vi "Get Visible (Label).vi"(8 "error in (no error)":errorcluster, 10 "Label":string, 11 "IObject in":refnum<class "IObject.lvclass">) -> (0 "error out":errorcluster, 1 "Match?":bool, 2 "Visible?":bool, 3 "IObject out":refnum<class "IObject.lvclass">, 4 "Item visible?":bool)   [LabVIEW 2021, in "IObject.lvclass"]
uses:
  IObject.lvclass
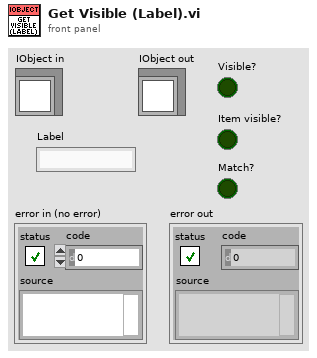
[diagram p1: front panel]
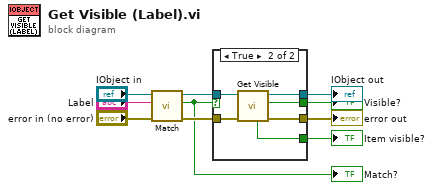
[diagram p0: block diagram]
diagram:
  n1 = call "Match.vi"("error in (no error)"="error in (no error)", "Label"="Label", "MMI Scaling in"="IObject in") -> ("error out"=w7:errorcluster, "Match?"=w1:bool, "MMI Scaling out"=w5:refnum<class "IObject.lvclass">)  [unwired: 6 in]
  "Match?" <- w1
  n2 = case shown="True" w1 {
    tunnel: w7 -> [w11 w18]
    tunnel: [w11 w17] -> w6
    tunnel: w5 -> [w12 w16]
    tunnel: [w12 w15] -> w4
    tunnel: [_ w14] -> w3
    tunnel: [_ w13] -> w2
    frame False {
    }
    frame True {
      n3 = call-dynamic "Get Visible.vi"("error in (no error)"=w18, "IObject in"=w16) -> ("error out"=w17:errorcluster, "Visible?"=w14:bool, "IObject out"=w15:refnum<class "IObject.lvclass">, "Item visible?"=w13:bool)  [unwired: 6 in]
    }
  }
  "error out" <- w6
  "IObject out" <- w4
  "Visible?" <- w3
  "Item visible?" <- w2
